vi "fg_l3_config.vi"() -> (0 "runtime_command":string, 1 "runtime_address":string, 2 "display_name":string, 3 "registry_key":string)   [LabVIEW 2015, in "lv-builder-l3.lvlib"]
uses:
  lv-builder-l3.lvlib
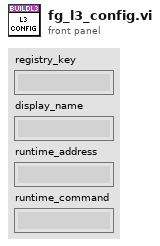
[diagram p1: front panel]
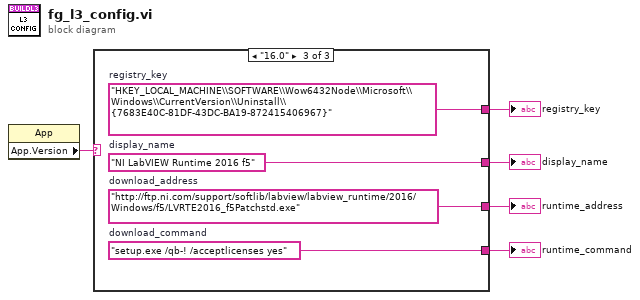
[diagram p0: block diagram]
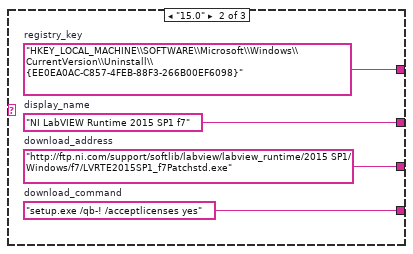
[diagram p3: hidden frame]
diagram:
  n1 = property class="App"() -> ("App.Version"=w5:string)  [unwired: 2 in, 2 out]
  n2 = case shown="\"16.0\"" w5 {
    tunnel: [_ w9 w13] -> w4
    tunnel: [_ w6 w10] -> w1
    tunnel: [_ w7 w11] -> w2
    tunnel: [_ w8 w12] -> w3
    frame Default {
    }
    frame "15.0" {
      w6 = "setup.exe /qb-! /acceptlicenses yes"  # download_command
      w7 = "http://ftp.ni.com/support/softlib/labview/labview_runtime/2015 SP1/Windows/f7/LVRTE2015SP1_f7Patchstd.exe"  # download_address
      w8 = "NI LabVIEW Runtime 2015 SP1 f7"  # display_name
      w9 = "HKEY_LOCAL_MACHINE\\SOFTWARE\\Microsoft\\Windows\\CurrentVersion\\Uninstall\\{EE0EA0AC-C857-4FEB-88F3-266B00EF6098}"  # registry_key
    }
    frame "16.0" {
      w10 = "setup.exe /qb-! /acceptlicenses yes"  # download_command
      w11 = "http://ftp.ni.com/support/softlib/labview/labview_runtime/2016/Windows/f5/LVRTE2016_f5Patchstd.exe"  # download_address
      w12 = "NI LabVIEW Runtime 2016 f5"  # display_name
      w13 = "HKEY_LOCAL_MACHINE\\SOFTWARE\\Wow6432Node\\Microsoft\\Windows\\CurrentVersion\\Uninstall\\{7683E40C-81DF-43DC-BA19-872415406967}"  # registry_key
    }
  }
  "registry_key" <- w4
  "display_name" <- w3
  "runtime_address" <- w2
  "runtime_command" <- w1
